vi "Example_SingleMeasurement.vi"(1 "base path":path=path "C:/Users/CFRFDA/Desktop/Labview Software/LQ_CO_RS485SensorCable_LabView_Support_32bit_2_D2/Support", 2 "COMPort":u16=19) -> (0 "MeasureResult Scaled":dbl)   [LabVIEW 2014]
uses:
  Sensirion_RS485SensorCable.llb/aResolution.ctl
  Sensirion_RS485SensorCable.llb/aHeaterMode.ctl
  Sensirion_RS485SensorCable.llb/aCalibField.ctl
  Sensirion_RS485SensorCable.llb/aLinearization.ctl
  Sensirion_RS485SensorCable.llb/aMeasureType.ctl
panel:
  out "aMeasureType 2":T1 items=["Flow", "Temperature", "Supply Voltage"]
  in  "aMeasureType":T1 items=["Flow", "Temperature", "Supply Voltage"]
  out "aFlowUnitString":string
  out "aScaleFactor":u16
  out "aLinearization 2":T2 items=["disabled", "enabled"]
  in  "aLinearization":T2=1 items=["disabled", "enabled"]
  out "aCalibField 2":T3 items=["4"=4, "3"=3, "2"=2, "1"=1, "0"=0]
  in  "aCalibField":T3 items=["4"=4, "3"=3, "2"=2, "1"=1, "0"=0]
  out "aHeaterMode 2":T4 items=["always off", "always on", "only on for measurement"]
  in  "aHeaterMode":T4=1 items=["always off", "always on", "only on for measurement"]
  out "aResolution 2":T5 items=["16"=16, "15"=15, "14"=14, "13"=13, "12"=12, "11"=11, "10"=10, "9"=9]
  in  "aResolution":T5=16 items=["16"=16, "15"=15, "14"=14, "13"=13, "12"=12, "11"=11, "10"=10, "9"=9]
  out "aMeasureResult unscaled":i32
  in  "aSlaveAdr":u8
  # "Communication Settings"
  # "Measurement Settings"
  # "Measurement Settings Read"
  # "Measurement Information"
  # "Measurement Result"
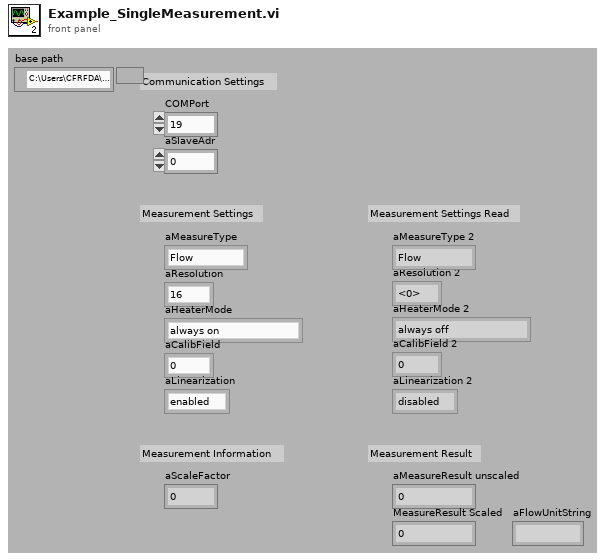
[diagram p1: front panel]
types:
  T1 = typedef "aMeasureType.ctl" = u8
  T2 = typedef "aLinearization.ctl" = u8
  T3 = typedef "aCalibField.ctl" = u8
  T4 = typedef "aHeaterMode.ctl" = u8
  T5 = typedef "aResolution.ctl" = u8
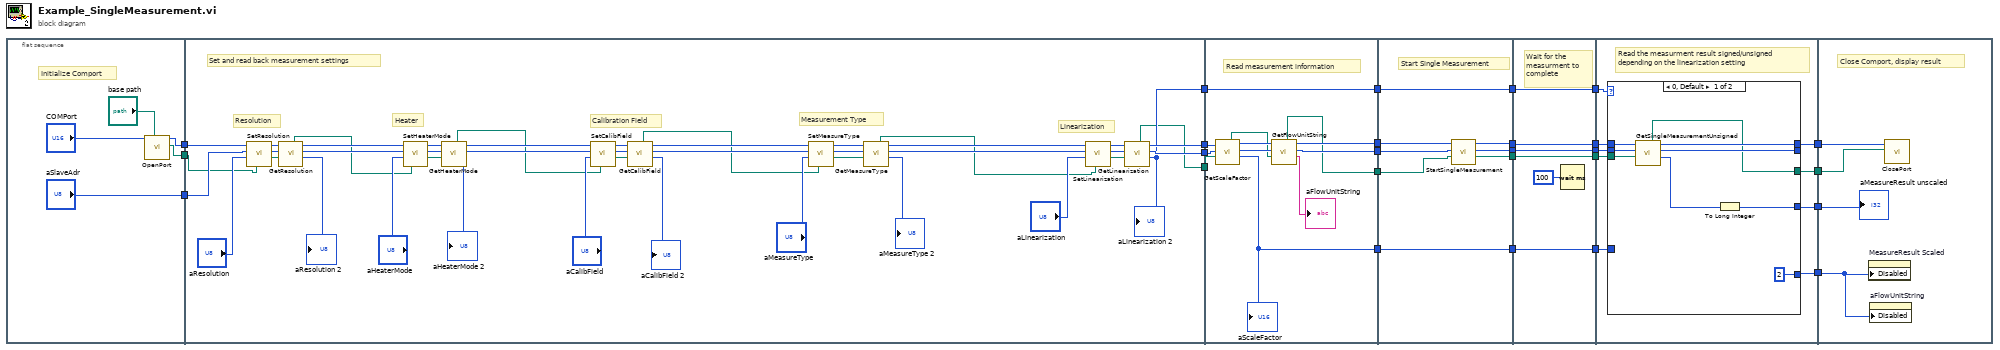
[diagram p0: block diagram]
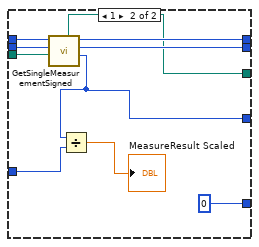
[diagram p2: hidden frame]
diagram:
  n1 = flat-sequence {
    tunnel: [w30] -> w8
    tunnel: ["aSlaveAdr"] -> w7
    tunnel: [w27] -> w6
    tunnel: [w47] -> w22
    tunnel: [w46] -> w21
    tunnel: [w45] -> w9
    tunnel: w8 -> [w44]
    tunnel: w7 -> [w43]
    tunnel: w6 -> [w42]
    tunnel: [w32] -> w5
    tunnel: w22 -> [w83]
    tunnel: w21 -> [w82]
    tunnel: [w81] -> w20
    tunnel: [w80] -> w19
    tunnel: [w79] -> w13
    tunnel: [w78] -> w10
    tunnel: w9 -> [w78]
    tunnel: w5 -> [w77]
    tunnel: [w75] -> w4
    tunnel: [w92] -> w24
    tunnel: [w91] -> w23
    tunnel: w20 -> [w94]
    tunnel: w19 -> [w93]
    tunnel: [w90] -> w14
    tunnel: w13 -> [w90]
    tunnel: [w89] -> w11
    tunnel: w10 -> [w89]
    tunnel: w4 -> [w88]
    tunnel: [w87] -> w2
    tunnel: [w99] -> w26
    tunnel: [w98] -> w25
    tunnel: w24 -> [w99]
    tunnel: w23 -> [w98]
    tunnel: [w97] -> w15
    tunnel: w14 -> [w97]
    tunnel: [w96] -> w12
    tunnel: w11 -> [w96]
    tunnel: [w95] -> w3
    tunnel: w2 -> [w95]
    tunnel: w26 -> [w109]
    tunnel: w25 -> [w108]
    tunnel: [w107] -> w18
    tunnel: [w106] -> w17
    tunnel: [w105] -> w16
    tunnel: w15 -> [w104]
    tunnel: w12 -> [w103]
    tunnel: w3 -> [w102]
    tunnel: [w101] -> w1
    tunnel: w18 -> [w132]
    tunnel: w17 -> [w131]
    tunnel: w16 -> [w130]
    tunnel: w1 -> [w129]
    frame #0 {
      # "Initialize Comport"
      n2 = call "OpenPort.vi"("base path"="base path", "COMPort"="COMPort") -> ("base path 2"=w27:path, "aPortHandle"=w30:u32)  [unwired: 7 in, 1 out]
    }
    frame #1 {
      # "Linearization"
      # "Measurement Type"
      # "Calibration Field"
      # "Heater"
      # "Resolution"
      # "Set and read back measurement settings"
      n3 = call "SetResolution.vi"("base path"=w42, "aResolution"="aResolution", "aSlaveAdr"=w43, "aPortHandle"=w44) -> ("base path 2"=w41:path, "aSlaveAdr"=w50:u8, "aPortHandle"=w49:u32)  [unwired: 4 in, 1 out]
      n4 = call "GetResolution.vi"("base path"=w41, "aSlaveAdr"=w50, "aPortHandle"=w49) -> ("aResolution"=→"aResolution 2":T5, "aSlaveAdr"=w54:u8, "aPortHandle"=w52:u32, "base path 2"=w40:path)  [unwired: 4 in, 1 out]
      n5 = call "SetHeaterMode.vi"("base path"=w40, "aHeaterMode"="aHeaterMode", "aSlaveAdr"=w54, "aPortHandle"=w52) -> ("base path 2"=w39:path, "aSlaveAdr"=w55:u8, "aPortHandle"=w53:u32)  [unwired: 4 in, 1 out]
      n6 = call "GetHeaterMode.vi"("base path"=w39, "aSlaveAdr"=w55, "aPortHandle"=w53) -> ("aHeaterMode"=→"aHeaterMode 2":T4, "aSlaveAdr"=w59:u8, "aPortHandle"=w58:u32, "base path 2"=w38:path)  [unwired: 4 in, 1 out]
      n7 = call "SetCalibField.vi"("base path"=w38, "aCalibField"="aCalibField", "aSlaveAdr"=w59, "aPortHandle"=w58) -> ("base path 2"=w37:path, "aSlaveAdr"=w62:u8, "aPortHandle"=w61:u32)  [unwired: 4 in, 1 out]
      n8 = call "GetCalibField.vi"("base path"=w37, "aSlaveAdr"=w62, "aPortHandle"=w61) -> ("aCalibField"=→"aCalibField 2":T3, "aSlaveAdr"=w68:u8, "aPortHandle"=w67:u32, "base path 2"=w36:path)  [unwired: 4 in, 1 out]
      n9 = call "SetMeasureType.vi"("base path"=w36, "aMeasureType"="aMeasureType", "aSlaveAdr"=w68, "aPortHandle"=w67) -> ("base path 2"=w35:path, "aSlaveAdr"=w71:u8, "aPortHandle"=w70:u32)  [unwired: 4 in, 1 out]
      n10 = call "GetMeasureType.vi"("base path"=w35, "aSlaveAdr"=w71, "aPortHandle"=w70) -> ("aMeasureType"=→"aMeasureType 2":T1, "aSlaveAdr"=w74:u8, "aPortHandle"=w73:u32, "base path 2"=w34:path)  [unwired: 4 in, 1 out]
      n11 = call "SetLinearization.vi"("base path"=w34, "aLinearization"="aLinearization", "aSlaveAdr"=w74, "aPortHandle"=w73) -> ("base path 2"=w33:path, "aSlaveAdr"=w66:u8, "aPortHandle"=w65:u32)  [unwired: 4 in, 1 out]
      n12 = call "GetLinearization.vi"("base path"=w33, "aSlaveAdr"=w66, "aPortHandle"=w65) -> ("aLinearization"=w45:T2, "aSlaveAdr"=w46:u8, "aPortHandle"=w47:u32, "base path 2"=w32:path)  [unwired: 4 in, 1 out]
      "aLinearization 2" <- w45
    }
    frame #2 {
      # "Read measurement information"
      n13 = call "GetScaleFactor.vi"("base path"=w77, "aSlaveAdr"=w82, "aPortHandle"=w83) -> ("aScaleFactor"=w79:u16, "aSlaveAdr"=w85:u8, "aPortHandle"=w84:u32, "base path 2"=w76:path)  [unwired: 4 in, 1 out]
      "aScaleFactor" <- w79
      n14 = call "GetFlowUnitString.vi"("base path"=w76, "aSlaveAdr"=w85, "aPortHandle"=w84) -> ("aFlowUnitString"=→"aFlowUnitString":string, "aSlaveAdr"=w80:u8, "aPortHandle"=w81:u32, "base path 2"=w75:path)  [unwired: 4 in, 1 out]
    }
    frame #3 {
      # "Start Single Measurement"
      n15 = call "StartSingleMeasurement.vi"("base path"=w88, "aSlaveAdr"=w93, "aPortHandle"=w94) -> ("base path 2"=w87:path, "aSlaveAdr"=w91:u8, "aPortHandle"=w92:u32)  [unwired: 5 in, 1 out]
    }
    frame #4 {
      # "Wait for the\nmeasurment to\ncomplete"
      n16 = Wait (ms)(milliseconds to wait=u32 100) -> ()  [unwired: 1 out]
    }
    frame #5 {
      # "Read the measurment result signed/unsigned\ndepending on the linearization setting"
      n17 = case shown="0, Default" w103 {
        tunnel: [w118 w126] -> w106
        tunnel: w109 -> [w117 w128]
        tunnel: w108 -> [w116 w127]
        tunnel: [w115 w125] -> _
        tunnel: w104 -> [_ w124]
        tunnel: [w113 w122] -> w107
        tunnel: [u8 2 ("Disabled") u8 0 ("Disabled")] -> w105
        tunnel: w102 -> [w111 w120]
        tunnel: [w110 w119] -> w101
        frame 0, Default {
          n18 = call "GetSingleMeasurementUnsigned.vi"("base path"=w111, "aSlaveAdr"=w116, "aPortHandle"=w117) -> ("aMeasureResult"=w114:u16, "aSlaveAdr"=w115:u8, "aPortHandle"=w118:u32, "base path 2"=w110:path)  [unwired: 4 in, 1 out]
          n19 = To Long Integer(number=w114) -> (32bit integer=w113:i32)
        }
        frame 1 {
          n20 = call "GetSingleMeasurementSigned.vi"("base path"=w120, "aSlaveAdr"=w127, "aPortHandle"=w128) -> ("aMeasureResult"=w122:i16, "aSlaveAdr"=w125:u8, "aPortHandle"=w126:u32, "base path 2"=w119:path)  [unwired: 4 in, 1 out]
          n21 = Divide(x=w122, y=w124) -> (x/y=→"MeasureResult Scaled":dbl)
        }
      }
    }
    frame #6 {
      # "Close Comport, display result"
      n22 = property on="MeasureResult Scaled" class="DigNum (strict)"("Disabled"=w130) -> ()  [unwired: 2 in, 2 out]
      n23 = property on="aFlowUnitString" class="Str"("Disabled"=w130) -> ()  [unwired: 2 in, 2 out]
      n24 = call "ClosePort.vi"("base path"=w129, "aPortHandle"=w131) -> ()  [unwired: 8 in, 2 out]
      "aMeasureResult unscaled" <- w132
    }
  }
